vi "Load Configuration.vi"(8 "error in":errorcluster) -> (0 "error out":errorcluster, 3 "Theme Config out":refnum<class "Theme Config.lvclass">)   [LabVIEW 2021, in "Theme Config.lvclass"]
doc: "Load the configuration from file; if it doesn't exist, go ahead and create it so it can be referenced in the future.\n\nThis will allow persistence of the Material File in the editor and the Last Theme Mod implemented.\n\n<b>Code Developed By:</b>\nDaniel Coons\nTechnology Service Corporation\nwww.tsc.com/atcs"
uses:
  Theme Config.lvclass
  C:/Program Files/National Instruments/LabVIEW 2026/vi.lib/JDP Science/JSONtext/Config Files/Config File.lvclass
  Theme Serializer/Theme Serializer.lvclass
  C:/Program Files/National Instruments/LabVIEW 2026/vi.lib/JDP Science/JSONtext/LVClass Serializer/JSONtext LVClass Serializer.lvclass
  Theme Config.lvclass/Theme Config.ctl
  <vilib>/JDP Science/JSONtext/Config Files/Config File.lvclass/Config File.ctl
  <vilib>/JDP Science/JSONtext/Config Files/Config File.lvclass
  <vilib>/JDP Science/JSONtext/JSONtext.lvlib
  3b317bd2-2840-4331-bfb7-99d377f3c52f.vi
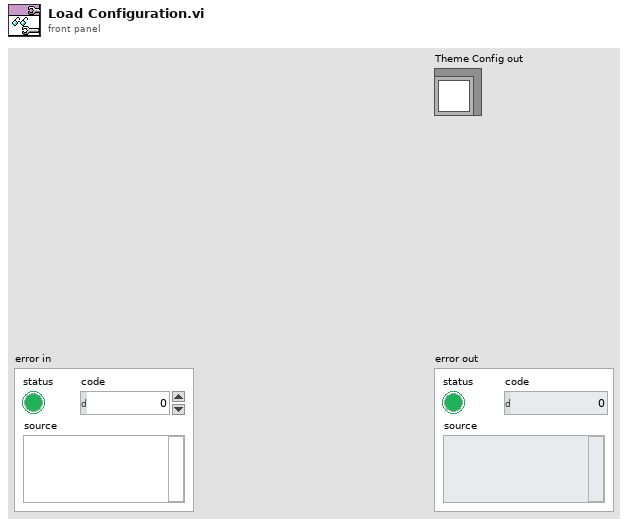
[diagram p1: front panel]
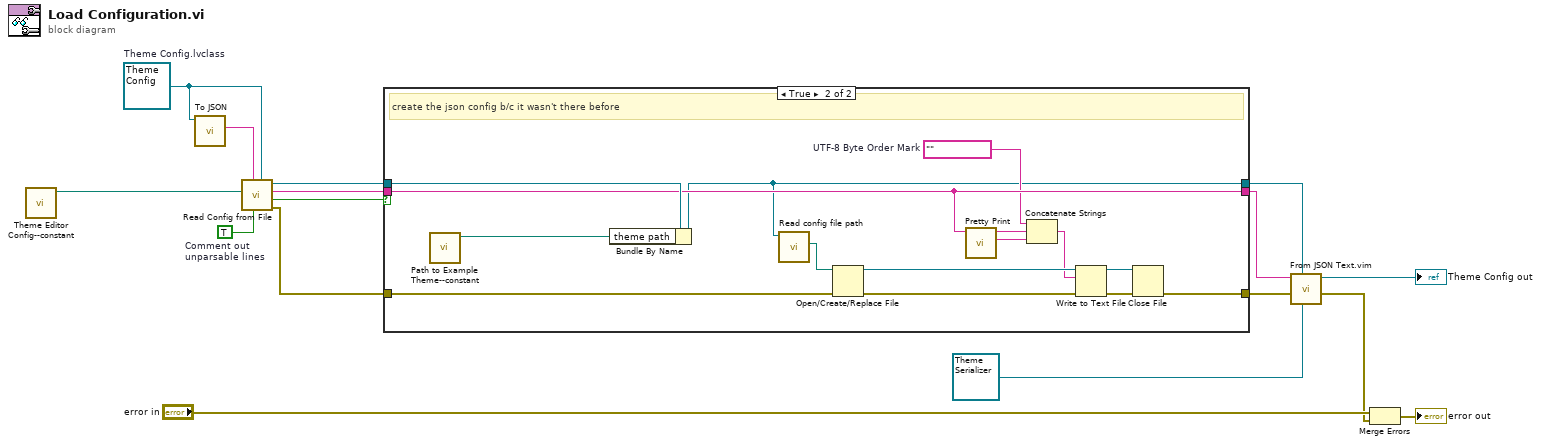
[diagram p0: block diagram]
diagram:
  w11 = TRUE  # Comment out unparsable lines
  w14 = refnum<class "Theme Config.lvclass"> refnum  # Theme Config.lvclass
  n1 = call "Theme Editor Config--constant.vi"() -> ("Button Editor Config"=w12:path)  [unwired: 11 in]
  n2 = call "To JSON.vi"("Theme Config in"=w14) -> ("JSON"=w13:string)  [unwired: 8 in, 2 out]
  n3 = call <vilib>:"Read Config from File.vi"("Config File (type)"=w14, "Comment out unparsable lines"=w11, "Template (JSON Object)"=w13, "config file path"=w12) -> ("error out"=w9:errorcluster, "Template Used (file missing or corrupted)"=w10:bool, "<JSON>Config"=w8:string, "Config File"=w7:refnum<class "Theme Config.lvclass">)  [unwired: 4 in]
  n4 = case shown="True" w10 {
    tunnel: w9 -> [w19 w34]
    tunnel: w8 -> [w18 w29]
    tunnel: w7 -> [w17 w33]
    tunnel: [w17 w21] -> w4
    tunnel: [w18 w29] -> w5
    tunnel: [w19 w22] -> w6
    frame False {
    }
    frame True {
      w26 = "﻿"  # UTF-8 Byte Order Mark
      # "create the json config b/c it wasn't there before"
      n5 = call "Path to Example Theme--constant.vi"() -> ("Path to Example Theme"=w20:path)  [unwired: 11 in]
      n6 = Bundle By Name(cluster=w33, "theme path"=w20) -> (w21:refnum<class "Theme Config.lvclass">)
      n7 = call <vilib>:"Read config file path.vi"("Config File in"=w21) -> ("config file path"=w32:path)  [unwired: 10 in]
      n8 = Open/Create/Replace File(file path (use dialog)=w32, error in=w34) -> (refnum out=w30:refnum<file>, error out=w31:errorcluster)  [unwired: 4 in, 1 out]
      n9 = call <vilib>:"Pretty Print.vi"("JSON"=w29) -> ("Rest of Input String"=w28:string, "<JSON>"=w27:string)  [unwired: 8 in, 1 out]
      n10 = Concatenate Strings(w26, w27, w28) -> (w25:string)
      n11 = Write to Text File(file (use dialog)=w30, text=w25, error in=w31) -> (refnum out=w23:refnum<file>, error out=w24:errorcluster)  [unwired: 1 in, 1 out]
      n12 = Close File(refnum=w23, error in=w24) -> (error out=w22:errorcluster)  [unwired: 1 out]
    }
  }
  n13 = call "From JSON Text.vim"("LVClass Serializer"=refnum<class "Theme Serializer.lvclass"> refnum ("Theme Serializer.lvclass"), "Data Type and Default Value"=w4, "error in (no error)"=w6, "JSON"=w5) -> ("error out"=w2:errorcluster, "Data out"=→"Theme Config out":refnum<class "Theme Config.lvclass">)  [unwired: 6 in]
  n14 = Merge Errors("error in", w2) -> (→"error out":errorcluster)
